vi "Detector Process File.vi"(8 "error in (no error)":errorcluster, 9 "Observation":T1={"Priority"=0, "ID"="", "Observer"="", "Obj Name"="", "Obj Type"="", "RA and DEC String"={"RA"="HH:MM:SS.nnn", "DEC"="DEG:arcmin:arcsec.nn"}, "Filter Wheel 1"="", "Filter Wheel 2"="", "Integration Time"=0.0, "Observation Status"=enum."Error", "Offsets"={"RA"=0.0, "DEC"=0.0, "ROT"=0.0}, "Images"=0, "Dither Options"={"Dither"=enum."None", "Dither Radius"=0.0, "Dither Points"=0, "Dither Phase"=0.0}, "Comment 1"="", "Comment 2"=""}, 10 "Detector Config":T6={"Detector"=0, "Offsets"=[[0, 0, 0, 0, 0, 0, 0, 0, 0, 0, 0, 0, 0, 0, 0, 0, 0, 0, 0, 0, 0, 0, 0, 0, 0, 0, 0, 0, 0, 0, 0, 0]], "Detector Computer"={"Machine"="192.168.121.11", "Password"="rSL!nux23456", "FITS File Path"="", "Port"=44444, "Header Path"="", "Name"=""}, "FITS hdr template0"=path "", "FITS hdr template1"=path "", "FITS Data File Path"=path "", "FITS Detector Settings"={"Exp Time Short"=0.0, "# of Frames"=0.0, "Exp Time Long"=0.0, "# of Groups"=0.0, "Object Name"="", "Object"="", "Obs Type"="", "Image Type"="", "Observer"="", "Observer Affiliation"=""}, "Sim Folder"=path "", "Integration Mode"=enum."SSR", "Integration Time"=0.0, "Frame Int Time"=0.0} {"Offsets" format="%04x"; "Detector" items=["0", "1", "2"]}, 11 "Image":T10) -> (0 "error out":errorcluster, 3 "FITS file":path)   [LabVIEW 2024]
uses:
  Detector Image typedef cluster.ctl
  RIMAS Detector Config.ctl
  RIMAS Detector Server Config.ctl
  RIMAS Observation Config.ctl
  Detector enum Detector Integration Mode.ctl
  typedefs/CC cluster Observation.ctl
  Observation Queue/CC enum Observation Status.ctl
  Telescope/CC cluster Telescope Offsets.ctl
  typedefs/CC cluster Observation Dither Options.ctl
  typedefs/CC enum Dither Selection.ctl
  gfitsio/gfitsio-write-key-integer.vi
  gfitsio/gfitsio-write-key-string.vi
  gfitsio/gfitsio-write-key-double.vi
  gfitsio/gfitsio.lvlib
  PRIME Detector.lvclass
  Detector Class.lvclass
panel:
  # "sec"
  # "sec"
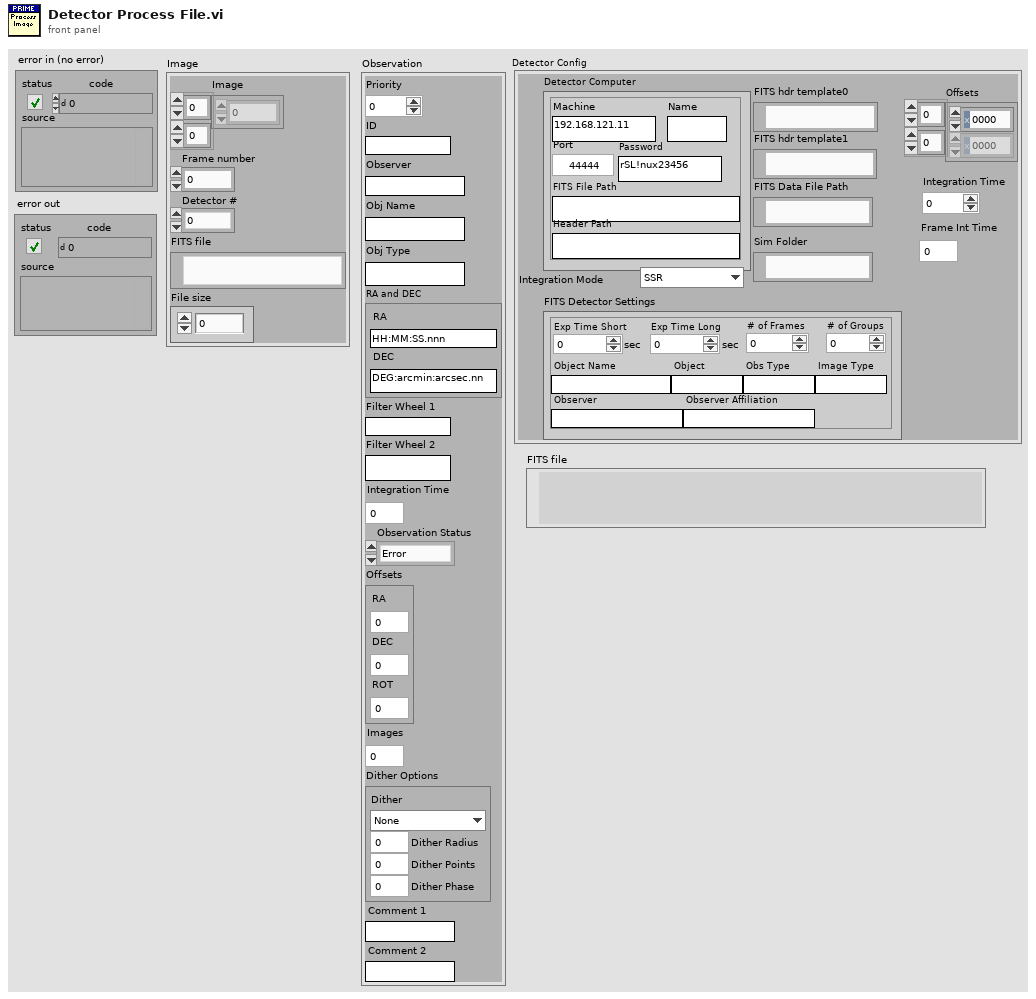
[diagram p1: front panel]
types:
  T1 = typedef "CC cluster Observation.ctl" = cluster{"Priority":i32, "ID":string, "Observer":string, "Obj Name":string, "Obj Type":string, "RA and DEC String":cluster{"RA":string, "DEC":string}, "Filter Wheel 1":string, "Filter Wheel 2":string, "Integration Time":dbl, "Observation Status":T2, "Offsets":T3, "Images":i32, "Dither Options":T4, "Comment 1":string, "Comment 2":string}
  T2 = typedef "CC enum Observation Status.ctl" = enum16{"Ready", "Running", "Done", "Error"}
  T3 = typedef "CC cluster Telescope Offsets.ctl" = cluster{"RA":dbl, "DEC":dbl, "ROT":dbl}
  T4 = typedef "CC cluster Observation Dither Options.ctl" = cluster{"Dither":T5, "Dither Radius":dbl, "Dither Points":i32, "Dither Phase":dbl}
  T5 = typedef "CC enum Dither Selection.ctl" = enum16{"None", "Circle", "Random"}
  T6 = typedef "RIMAS Detector Config.ctl" = cluster{"Detector":u16, "Offsets":u16[][], "Detector Computer":T7, "FITS hdr template0":path, "FITS hdr template1":path, "FITS Data File Path":path, "FITS Detector Settings":T8, "Sim Folder":path, "Integration Mode":T9, "Integration Time":dbl, "Frame Int Time":dbl}
  T7 = typedef "RIMAS Detector Server Config.ctl" = cluster{"Machine":string, "Password":string, "FITS File Path":string, "Port":u16, "Header Path":string, "Name":string}
  T8 = typedef "RIMAS Observation Config.ctl" = cluster{"Exp Time Short":dbl, "# of Frames":dbl, "Exp Time Long":dbl, "# of Groups":dbl, "Object Name":string, "Object":string, "Obs Type":string, "Image Type":string, "Observer":string, "Observer Affiliation":string}
  T9 = typedef "Detector enum Detector Integration Mode.ctl" = enum16{"SSR", "CDS", "MEAN", "MEDIAN", "MODE", "MIIN", "MAX"}
  T10 = typedef "Detector Class.lvclass/Detector Image typedef cluster.ctl" = cluster{"Image":sgl[][], "Frame number":i32, "Detector #":u16, "FITS file":path, "File size":i64}
  T11 = typedef "FITS cluster Header Row.ctl" = cluster{"Field Name":string, "Type":T12, "Value":string, "Comment":string, "Units":string}
  T12 = typedef "FITS enum Data Type.ctl" = enum16{"String", "Integer", "Float"}
  T13 = typedef "gfitsio.lvlib/gfitsio-refnum.ctl" = u64
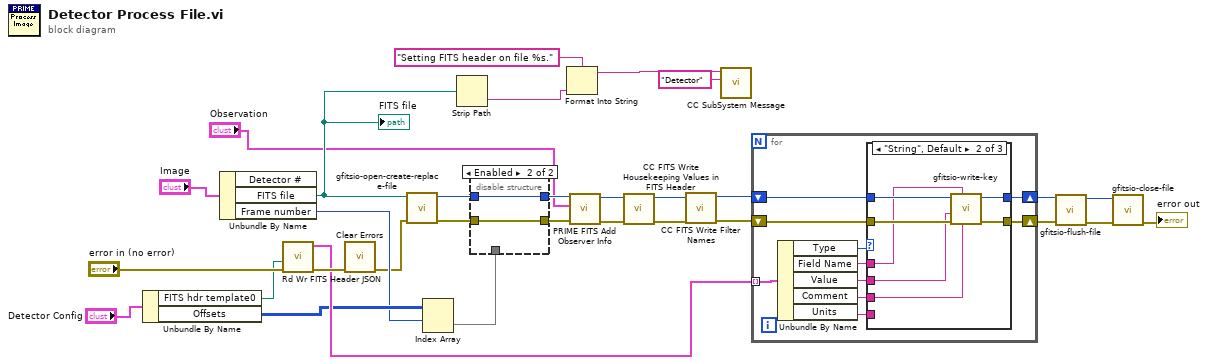
[diagram p0: block diagram]
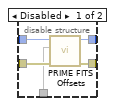
[diagram p2: hidden frame]
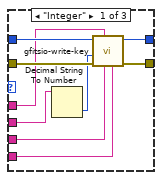
[diagram p3: hidden frame]
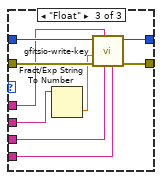
[diagram p4: hidden frame]
diagram:
  n1 = Unbundle By Name("Detector Config") -> ("FITS hdr template0"=w2:path, "Offsets"=w6:u16[][])
  n2 = Unbundle By Name("Image") -> ("FITS file"=w15:path, "Frame number"=w5:i32)  [unwired: 1 out]
  "FITS file" <- w15
  n3 = call "Rd Wr FITS Header JSON.vi"("error in (no error)"="error in (no error)", "FITS Template"=w2) -> ("error out"=w9:errorcluster, "FITS Hdr Rows"=w7:T11[])  [unwired: 8 in]
  n4 = call <vilib>:"Clear Errors.vi"("error in (no error)"=w9) -> ("error out"=w1:errorcluster)  [unwired: 5 in, 1 out]
  n5 = call "gfitsio-open-create-replace-file.vi"("error in (no error)"=w1, "file path (dialog if empty)"=w15) -> ("error out"=w31:errorcluster, "gfits refnum"=w30:T13)  [unwired: 7 in, 1 out]
  n6 = Index Array(array=w6, index (row)=w5) -> (element=w25:u16[])  [unwired: 1 in]
  n7 = Strip Path(path=w15) -> (name=w14:string)  [unwired: 1 out]
  n8 = disable-structure shown="Enabled" {
    disable-tunnel: w31 -> [w36 w37]
    disable-tunnel: w30 -> [w35 w38]
    disable-tunnel: [w34 w38] -> w29
    disable-tunnel: [w33 w37] -> w28
    disable-tunnel: w25 -> [w32 _]
    frame Disabled {
      n9 = call "PRIME FITS Offsets.vi"("error in (no error)"=w36, "Offsets"=w32, "gfits refnum"=w35) -> ("error out"=w33:errorcluster, "gfits refnum out"=w34:T13)  [unwired: 7 in]
    }
    frame Enabled {
    }
  }
  n10 = Format Into String(format string="Setting FITS header on file %s.", w14) -> (resulting string=w12:string)  [unwired: 2 in, 1 out]
  n11 = call "PRIME FITS Add Observer Info.vi"("Error In"=w28, "Observation"="Observation", "gfits refnum"=w29) -> ("Error Out"=w22:errorcluster, "dup gfits refnum"=w21:T13)  [unwired: 7 in]
  n12 = call "CC FITS Write Housekeeping Values in FITS Header.vi"("error in (no error)"=w22, "gfits refnum"=w21) -> ("error out"=w20:errorcluster, "dup gfits refnum"=w18:T13)  [unwired: 8 in]
  n13 = call "CC FITS Write Filter Names.vi"("error in (no error)"=w20, "gfits refnum"=w18) -> ("error out"=w19:errorcluster, "dup gfits refnum"=w17:T13)  [unwired: 8 in]
  n14 = call "CC SubSystem Message.vi"("Subsystem"="Detector", "Message"=w12) -> ()  [unwired: 9 in, 1 out]
  n15 = for {
    shift-right: [w45] -> w24
    shift-left: w17 -> [w47]
    shift-right: [w44] -> w23
    shift-left: w19 -> [w46]
    tunnel: w7 -> [w48] mode=indexing
    n16 = Unbundle By Name(w48) -> ("Type"=w43:T12, "Field Name"=w42:string, "Value"=w40:string, "Comment"=w41:string, "Units"=w39:string)
    n17 = case shown="\"String\", Default" w43 {
      tunnel: w47 -> [w57 w64 w73]
      tunnel: w46 -> [w56 w63 w72]
      tunnel: [w55 w62 w71] -> w45
      tunnel: [w54 w61 w70] -> w44
      tunnel: w42 -> [w53 w60 w69]
      tunnel: w41 -> [w52 w59 w68]
      tunnel: w40 -> [w51 w58 w67]
      tunnel: w39 -> [w49 _ w65]
      frame "Integer" {
        n18 = Decimal String To Number(string=w51) -> (number=w50:i32)  [unwired: 2 in, 1 out]
        n19 = call-poly "gfitsio-write-key.vi"("units"=w49, "comment"=w52, "keyname"=w53, "error in (no error)"=w56, "value"=w50, "gfits refnum"=w57) -> ("error out"=w54:errorcluster, "dup gfits refnum"=w55:T13)  [unwired: 4 in]
      }
      frame "String", Default {
        n20 = call-poly "gfitsio-write-key.vi"("comment"=w59, "keyname"=w60, "error in (no error)"=w63, "value"=w58, "gfits refnum"=w64) -> ("error out"=w61:errorcluster, "dup gfits refnum"=w62:T13)  [unwired: 5 in]
      }
      frame "Float" {
        n21 = Fract/Exp String To Number(string=w67) -> (number=w66:dbl)  [unwired: 3 in, 1 out]
        n22 = call-poly "gfitsio-write-key.vi"("units"=w65, "comment"=w68, "keyname"=w69, "error in (no error)"=w72, "value"=w66, "gfits refnum"=w73) -> ("error out"=w70:errorcluster, "dup gfits refnum"=w71:T13)  [unwired: 4 in]
      }
    }
  }
  n23 = call "gfitsio-flush-file.vi"("error in (no error)"=w23, "gfits refnum"=w24) -> ("error out"=w27:errorcluster, "dup gfits refnum"=w26:T13)  [unwired: 8 in]
  n24 = call "gfitsio-close-file.vi"("error in (no error)"=w27, "gfits refnum"=w26) -> ("error out"=→"error out":errorcluster)  [unwired: 8 in, 1 out]
